vi "testSumin.vi"() -> ()   [LabVIEW 2011]
uses:
  <vilib>/vision/Image Controls.llb/IMAQ Image.ctl
  <vilib>/vision/NI_Vision_Development_Module.lvlib
panel:
  out "*(类型 *) &x 2":T1
  out "*(类型 *) &x":string
  out "Image 2":T1(plugin-control)
  out "frame sum":T1[][](array[typedef])
  in  "sum rang 2":i32=120
  in  "sum rang 1":i32=40
  out "BlkFilePath":path
  out "stim":i32
  out "frame":i32
  out "Image":T1(plugin-control)
  out "Stimuli":i32
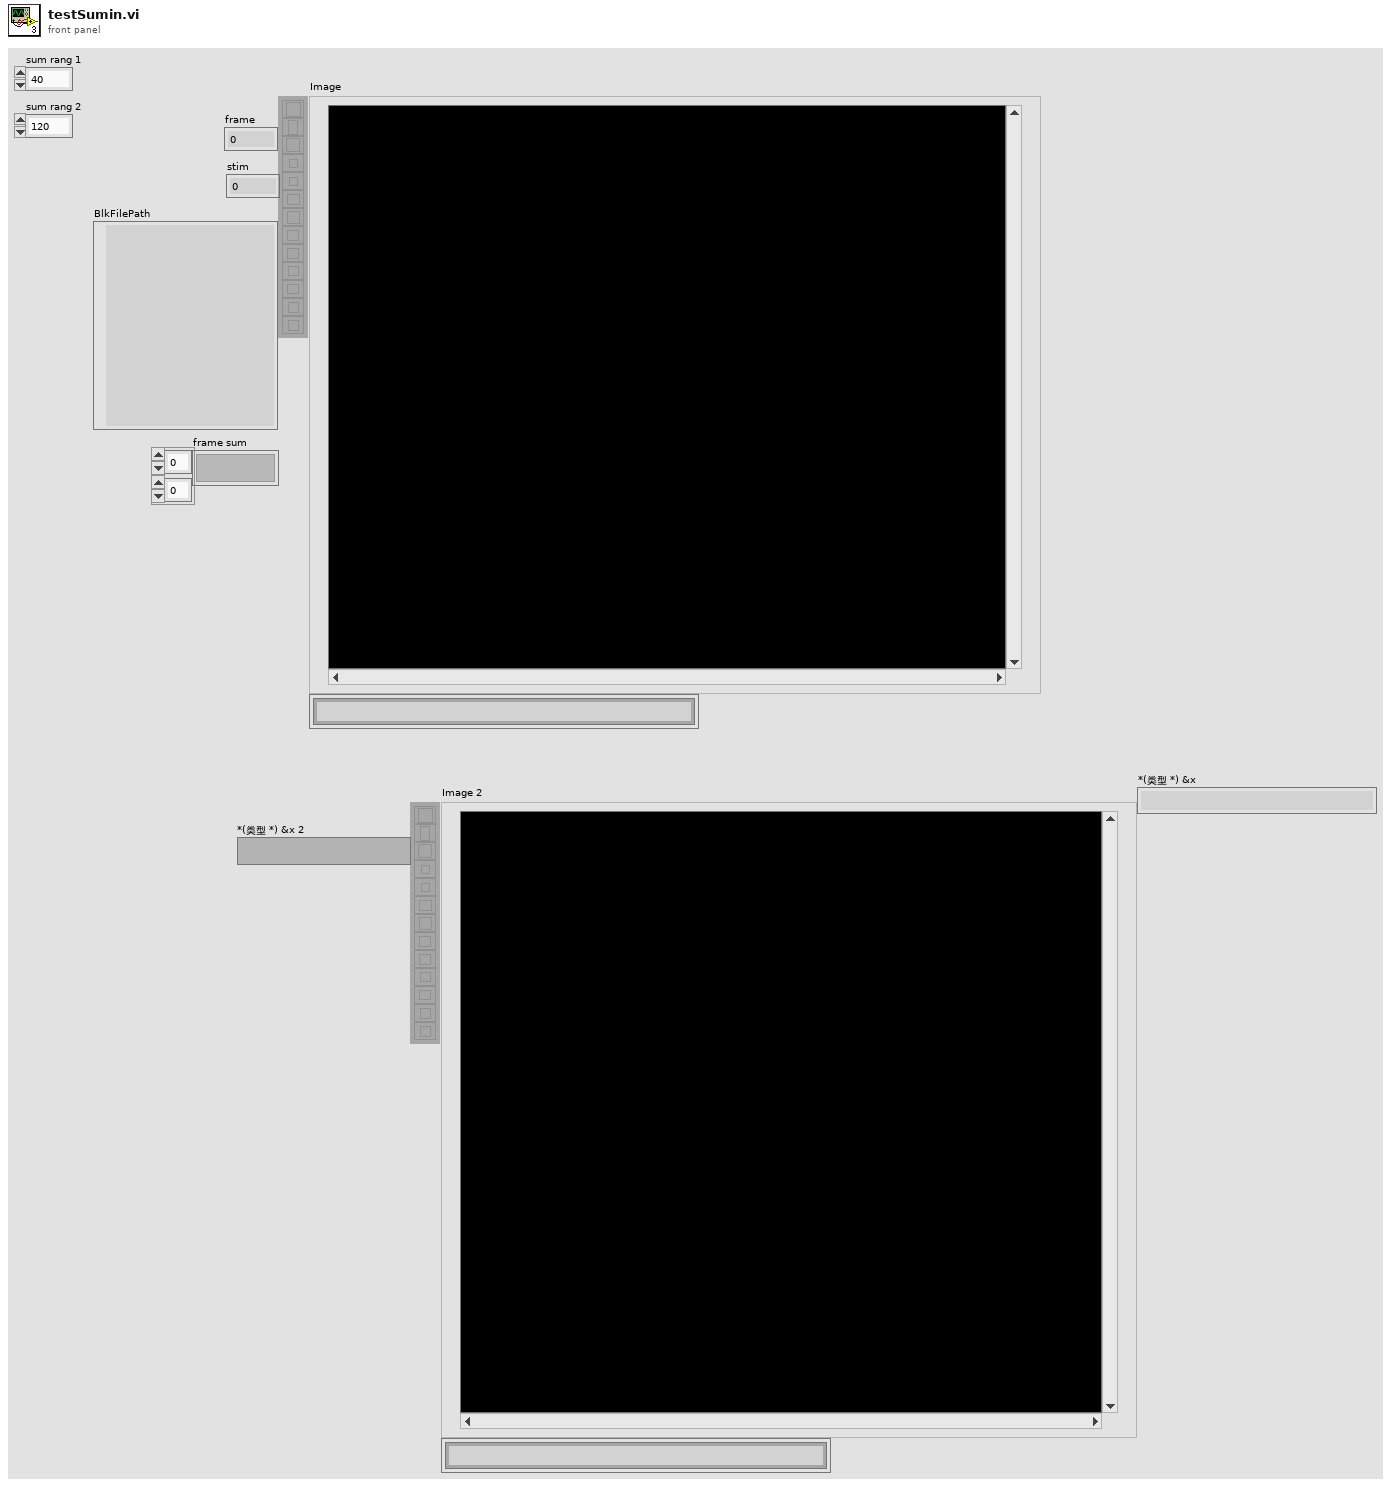
[diagram p1: front panel]
types:
  T1 = typedef "IMAQ Image.ctl" = refnum<image>
  T2 = typedef "Image Type" = u32
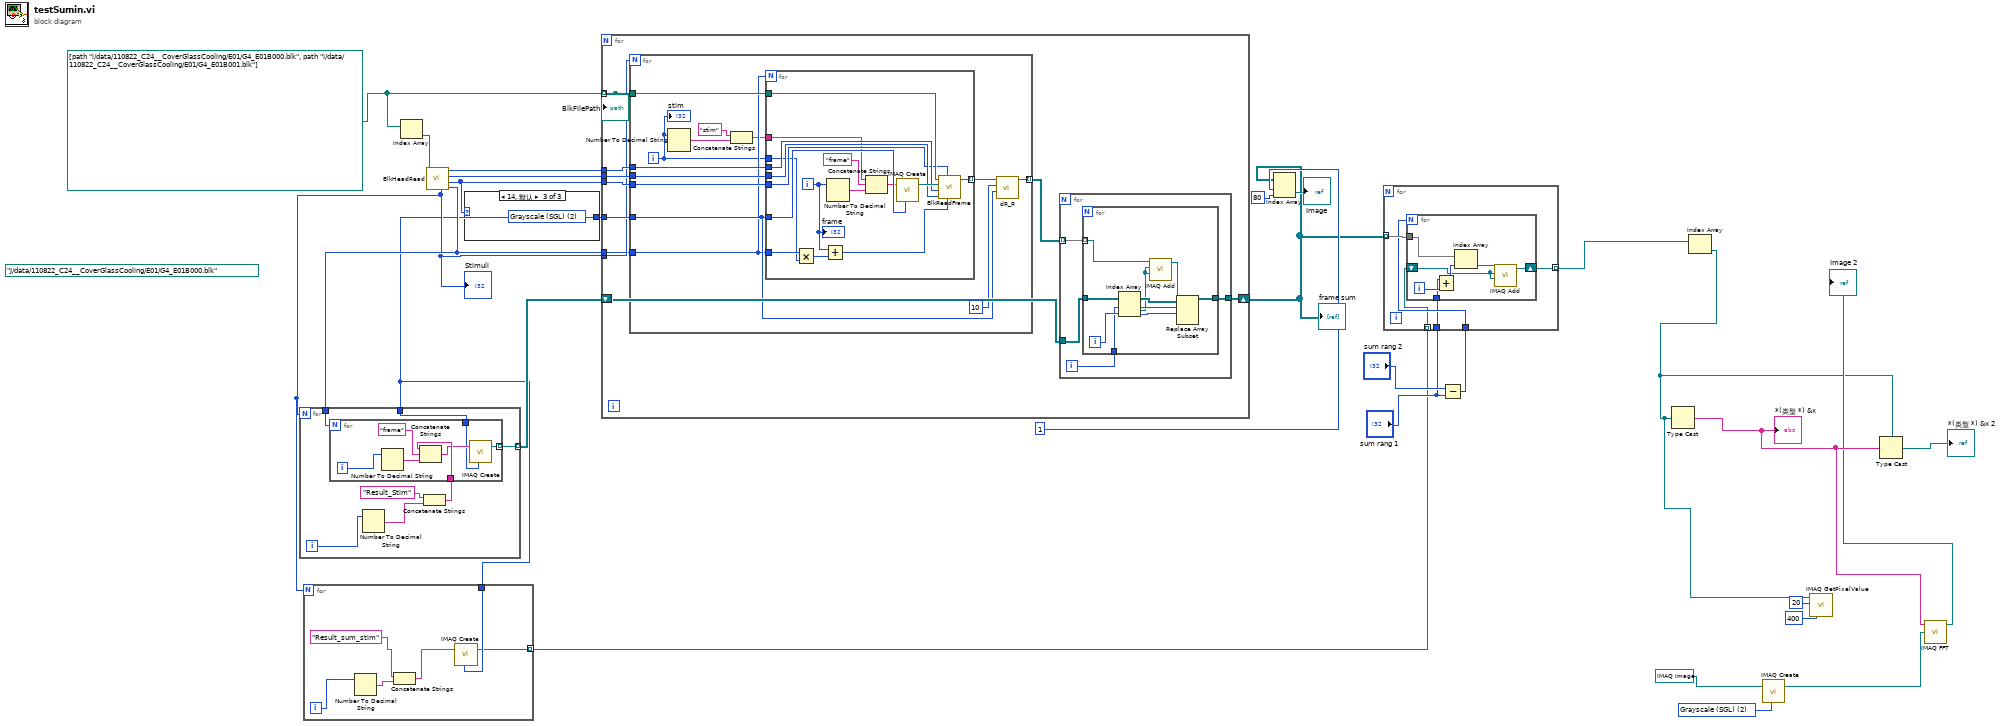
[diagram p0: block diagram]
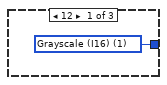
[diagram p2: hidden frame]
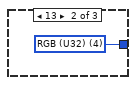
[diagram p3: hidden frame]
diagram:
  w4 = T2 2 items=["Grayscale (U8)", "Grayscale (I16)", "Grayscale (SGL)", "Complex (CSG)", "RGB (U32)", "HSL (U32)", "RGB (U64)", "Grayscale (U16)"] ("Image Type")
  (unwired) path "J:/data/110822_C24__CoverGlassCooling/E01/G4_E01B000.blk" ("BlkFilePath")
  w2 = path[] [path "i:/data/110822_C24__CoverGlassCooling/E01/G4_E01B000.blk", path "i:/data/110822_C24__CoverGlassCooling/E01/G4_E01B001.blk"]
  n1 = Index Array(array=w2) -> (element=w1:path)  [unwired: 1 in]
  n2 = call "BlkHeadRead.vi"("BlkFilePath"=w1) -> ("FramesPerStim"=w12:i32, "datatype"=w15:i32, "FrameHeight"=w16:i32, "FrameWidth"=w17:i32, "Stimuli"=w8:i32)  [unwired: 6 in]
  "Stimuli" <- w8
  n3 = case shown="14, 默认" w15 {
    tunnel: [w28 w29 w30] -> w7
    frame 12 {
      w28 = T2 1 items=["Grayscale (U8)", "Grayscale (I16)", "Grayscale (SGL)", "Complex (CSG)", "RGB (U32)", "HSL (U32)", "RGB (U64)", "Grayscale (U16)"] ("Image Type")
    }
    frame 13 {
      w29 = T2 4 items=["Grayscale (U8)", "Grayscale (I16)", "Grayscale (SGL)", "Complex (CSG)", "RGB (U32)", "HSL (U32)", "RGB (U64)", "Grayscale (U16)"] ("Image Type")
    }
    frame 14, Default {
      w30 = T2 2 items=["Grayscale (U8)", "Grayscale (I16)", "Grayscale (SGL)", "Complex (CSG)", "RGB (U32)", "HSL (U32)", "RGB (U64)", "Grayscale (U16)"] ("Image Type")
    }
  }
  n4 = for {
    N: w8 -> [_]
    tunnel: w7 -> [w33]
    tunnel: [w32] -> w14 mode=indexing
    tunnel: w12 -> [w31]
    i -> [w35]
    n5 = Number To Decimal String(number=w35) -> (decimal integer string=w36:string)  [unwired: 1 in]
    n6 = Concatenate Strings("Result_Stim" ("字符串"), w36) -> (w34:string)
    n7 = for {
      N: w31 -> [_]
      tunnel: w34 -> [w41]
      tunnel: w33 -> [w39]
      tunnel: [w38] -> w32 mode=indexing
      i -> [w42]
      n8 = Number To Decimal String(number=w42) -> (decimal integer string=w44:string)  [unwired: 1 in]
      n9 = Concatenate Strings(w41, "frame" ("字符串"), w44) -> (w40:string)
      n10 = call "IMAQ Create"("Image Name"=w40, "Image Type"=w39) -> ("New Image"=w38:T1)  [unwired: 3 in, 1 out]
    }
  }
  n11 = for {
    N: w8 -> [_]
    tunnel: w7 -> [w46]
    tunnel: [w45] -> w6 mode=indexing
    i -> [w50]
    n12 = Number To Decimal String(number=w50) -> (decimal integer string=w49:string)  [unwired: 1 in]
    n13 = Concatenate Strings("Result_sum_stim" ("字符串"), w49) -> (w47:string)
    n14 = call "IMAQ Create"("Image Name"=w47, "Image Type"=w46) -> ("New Image"=w45:T1)  [unwired: 3 in, 1 out]
  }
  n15 = for {
    tunnel: w17 -> [w60]
    tunnel: w16 -> [w59]
    tunnel: w15 -> [w58]
    tunnel: w2 -> [w57] mode=indexing
    tunnel: w7 -> [w56]
    tunnel: w8 -> [w55]
    tunnel: w12 -> [w54]
    shift-right: [w51] -> w13
    shift-left: w14 -> [w52]
    n16 = for {
      N: w55 -> [_]
      tunnel: w57 -> [w84]
      tunnel: w60 -> [w83]
      tunnel: w59 -> [w82]
      tunnel: w58 -> [w81]
      tunnel: w56 -> [w78]
      tunnel: w54 -> [w77]
      tunnel: [w76] -> w53 mode=indexing
      i -> [w75]
      n17 = Number To Decimal String(number=w75) -> (decimal integer string=w74:string)  [unwired: 1 in]
      n18 = Concatenate Strings("stim" ("字符串"), w74) -> (w72:string)
      n19 = for {
        N: w77 -> [_]
        tunnel: w78 -> [w98]
        tunnel: w84 -> [w96]
        tunnel: w83 -> [w94]
        tunnel: w82 -> [w93]
        tunnel: w81 -> [w92]
        tunnel: [w91] -> w80 mode=indexing
        tunnel: w75 -> [w89]
        tunnel: w77 -> [w90]
        tunnel: w72 -> [w85]
        i -> [w87]
        n20 = Multiply(x=w90, y=w89) -> (x*y=w88:i32)
        n21 = Add(x=w87, y=w88) -> (x+y=w86:i32)
        n22 = Number To Decimal String(number=w87) -> (decimal integer string=w99:string)  [unwired: 1 in]
        n23 = Concatenate Strings(w85, "frame" ("字符串"), w99) -> (w97:string)
        n24 = call "IMAQ Create"("Image Name"=w97, "Image Type"=w98) -> ("New Image"=w95:T1)  [unwired: 3 in, 1 out]
        n25 = call "BlkReadFrame.vi"("BlkFilePath"=w96, "datatype"=w92, "DST"=w95, "FrameWidth"=w94, "SkipFrame"=w86, "FrameHeight"=w93) -> ("Image out"=w91:T1)  [unwired: 2 in]
        "frame" <- w87
      }
      n26 = call "dR_R.vi"("Image Type"=w78, "initial frame NO."=10, "imaging input"=w80) -> ("imaging output"=w76:T1[])  [unwired: 8 in]
      "stim" <- w75
    }
    n27 = for {
      tunnel: w53 -> [w64] mode=indexing
      tunnel: w52 -> [w63]
      tunnel: [w61] -> w51
      i -> [w62]
      n28 = for {
        tunnel: w64 -> [w68] mode=indexing
        tunnel: w63 -> [w71]
        tunnel: w62 -> [w69]
        tunnel: [w67] -> w61
        i -> [w70]
        n29 = Index Array(array=w71, index (row)=w69, index (col)=w70) -> (element=w66:T1)
        n30 = call "IMAQ Add"("Image Src A"=w68, "Image Dst"=w66, "Image Src B"=w66) -> ("Image Dst Out"=w65:T1)  [unwired: 4 in, 1 out]
        n31 = Replace Array Subset(array=w71, new element=w65, index (row)=w69, index (col)=w70) -> (w67:T1[][])
      }
    }
    "BlkFilePath" <- w57
  }
  "frame sum" <- w13
  n32 = Index Array(array=w13, index (row)=1 ("索引"), index (col)=80 ("禁用的索引 (行)")) -> (element=→"Image":T1)
  n33 = Subtract(x="sum rang 2", y="sum rang 1") -> (x-y=w10:i32)
  n34 = for {
    tunnel: w13 -> [w105] mode=indexing
    tunnel: w10 -> [w104]
    tunnel: "sum rang 1" -> [w103]
    tunnel: w6 -> [w102] mode=indexing
    tunnel: [w101] -> w22 mode=indexing
    n35 = for {
      N: w104 -> [_]
      tunnel: w105 -> [w112]
      tunnel: w103 -> [w110]
      shift-right: [w106] -> w101
      shift-left: w102 -> [w107]
      i -> [w111]
      n36 = Add(x=w110, y=w111) -> (x+y=w109:i32)
      n37 = Index Array(array=w112, index=w109) -> (element=w108:T1)
      n38 = call "IMAQ Add"("Image Src A"=w108, "Image Dst"=w107, "Image Src B"=w107) -> ("Image Dst Out"=w106:T1)  [unwired: 4 in, 1 out]
    }
  }
  n39 = Index Array(array=w22) -> (element=w21:T1)  [unwired: 1 in]
  n40 = Type Cast(x=w21) -> (*(type *) &x=w24:string)  [unwired: 1 in]
  "*(类型 *) &x" <- w24
  n41 = call "IMAQ Create"("Image Name"=T1 refnum ("Image Dst"), "Image Type"=w4) -> ("New Image"=w3:T1)  [unwired: 3 in, 1 out]
  n42 = call "IMAQ GetPixelValue"("Image"=w21, "X Coordinate"=20, "Y Coordinate"=400) -> ()  [unwired: 3 in, 5 out]
  n43 = Type Cast(type=w21, x=w24) -> (*(type *) &x=→"*(类型 *) &x 2":T1)
  n44 = call "IMAQ FFT"("Image Dst"=w3, "Image Src"=w24) -> ("Image Dst Out"=→"Image 2":T1)  [unwired: 2 in, 1 out]
